vi "Next Step.vi"(8 "error in (no error)":errorcluster, 11 "Pulse Gen Scan.lvclass in":refnum<class "Pulse Gen Scan.lvclass">) -> (0 "error out":errorcluster, 1 "Current Step":u32, 2 "Current Position":dbl, 3 "Pulse Gen Scan.lvclass out":refnum<class "Pulse Gen Scan.lvclass">)   [LabVIEW 2012, in "Pulse Gen Scan.lvclass"]
uses:
  Pulse Gen Scan.lvclass
  Scanner/Scanner.lvclass
  Pulse Gen Scan.lvclass/Pulse Gen Scan.ctl
panel:
  out "time per bit":dbl[unit]
  out "Array of times used":dbl[unit][](array[numeric])
  out "Ch 2 Digital Waveform Graph":digitalwaveform(graph)
  out "Ch2 output string":string
  out "Ch1 output string":string
  out "Ch 1 Digital Waveform Graph":digitalwaveform(graph)
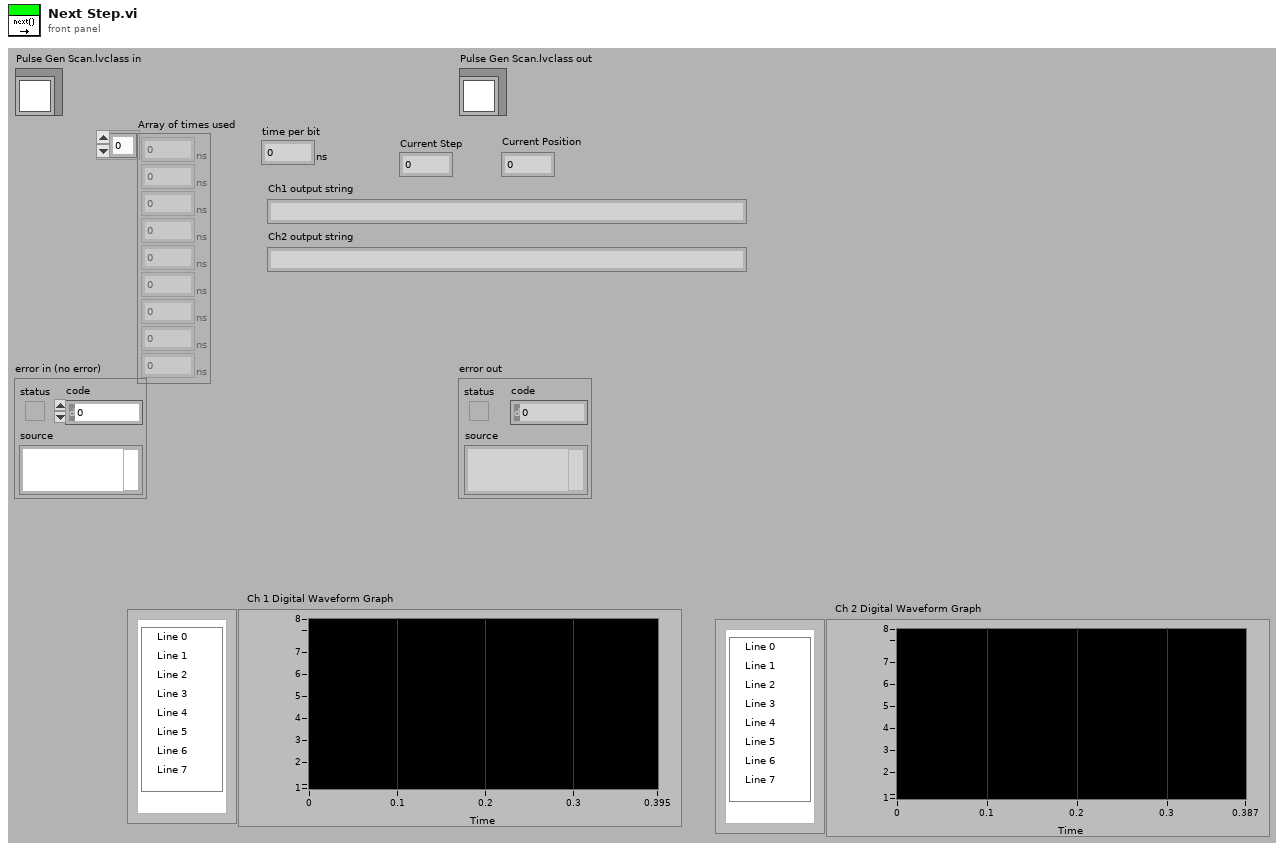
[diagram p1: front panel]
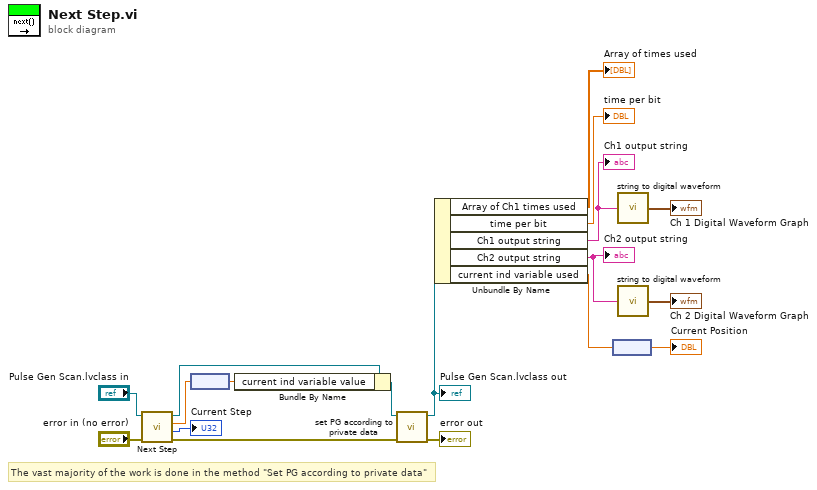
[diagram p0: block diagram]
diagram:
  # "The vast majority of the work is done in the method \"Set PG according to private data\""
  n1 = call-parent "Next Step.vi"("error in (no error)"="error in (no error)", "Scanner in"="Pulse Gen Scan.lvclass in") -> ("error out"=w1:errorcluster, "Current Step"=→"Current Step":u32, "Current Position"=w6:dbl, "Scanner out"=w4:refnum<class "Pulse Gen Scan.lvclass">)  [unwired: 6 out]
  n2 = node(w6) -> (w8:dbl[unit])
  n3 = Bundle By Name(cluster=w4, "current ind variable value"=w8) -> (w13:refnum<class "Pulse Gen Scan.lvclass">)
  n4 = call "set PG according to private data.vi"("error in (no error)"=w1, "Pulse Gen Scan in"=w13) -> ("error out"=→"error out":errorcluster, "Pulse Gen Scan out"=w5:refnum<class "Pulse Gen Scan.lvclass">)  [unwired: 8 in]
  "Pulse Gen Scan.lvclass out" <- w5
  n5 = Unbundle By Name(w5) -> ("Array of Ch1 times used"=→"Array of times used":dbl[unit][], "time per bit"=→"time per bit":dbl[unit], "Ch1 output string"=w12:string, "Ch2 output string"=w11:string, "current ind variable used"=w7:dbl[unit])
  "Ch1 output string" <- w12
  "Ch2 output string" <- w11
  n6 = node(w7) -> (→"Current Position":dbl)
  n7 = call "string to digital waveform.vi"("String"=w12) -> ("digital waveform"=→"Ch 1 Digital Waveform Graph":digitalwaveform)
  n8 = call "string to digital waveform.vi"("String"=w11) -> ("digital waveform"=→"Ch 2 Digital Waveform Graph":digitalwaveform)
